vi "stringToTimeStamp (SubVI).vi"(11 "strTime":string) -> (3 "Time Stamp":timestamp)   [LabVIEW 2017]
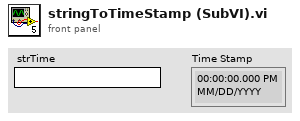
[diagram p1: front panel]
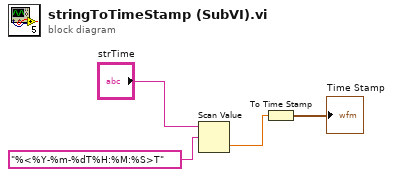
[diagram p0: block diagram]
diagram:
  n1 = Scan Value(string="strTime", format string="%<%Y-%m-%dT%H:%M:%S>T") -> (value=w3:dbl)  [unwired: 1 in, 1 out]
  n2 = To Time Stamp(1:w3) -> (0:→"Time Stamp":timestamp)
